vi "WPI_UtilitiesFRC LEDs.vi"(8 "error in (no error)":errorcluster, 10 "State":T1, 11 "LED Type":T2) -> (0 "error out":errorcluster, 3 "LED State":bool)   [LabVIEW 2019]
doc: "Sets the state, either on or off, of the USER1 LED or the FPGA LED on the CompactRIO device. You can define both the USER1 LED and the FPGA LED to meet the needs of your application.\n\nThis software is licensed. Open the labview\\readme\\WPI Robotics Library Open Source License.txt file for more information."
uses:
  <vilib>/Rock Robotics/SystemInterfaces/Utilities/FPGA_UtilitiesLED Source.ctl
  <vilib>/Rock Robotics/SystemInterfaces/Utilities/FPGA_UtilitiesLED State.ctl
  <vilib>/NI_Real-Time Target Support.lvlib
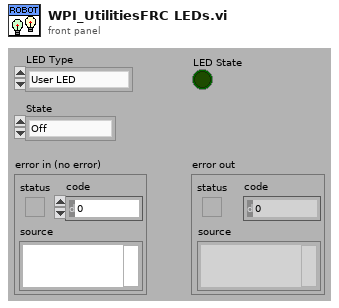
[diagram p1: front panel]
types:
  T1 = typedef "FPGA_UtilitiesLED State.ctl" = enum16{"Off", "On", "Toggle"}
  T2 = typedef "FPGA_UtilitiesLED Source.ctl" = enum16{"User LED", "FPGA LED"}
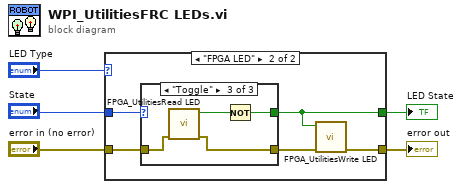
[diagram p0: block diagram]
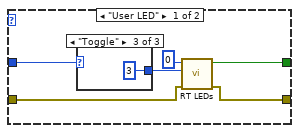
[diagram p2: hidden frame]
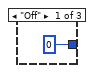
[diagram p3: hidden frame]
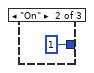
[diagram p4: hidden frame]
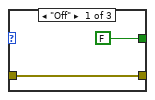
[diagram p5: hidden frame]
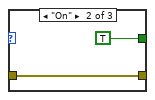
[diagram p6: hidden frame]
diagram:
  n1 = case shown="\"FPGA LED\"" "LED Type" {
    tunnel: "State" -> [w11 w19]
    tunnel: "error in (no error)" -> [w8 w16]
    tunnel: [w7 w18] -> w2
    tunnel: [w6 w17] -> w1
    frame "User LED" {
      n2 = case shown="\"Toggle\"" w11 {
        tunnel: [0 ("State") 1 ("State") 3 ("State")] -> w9
        frame "Off" {
        }
        frame "On" {
        }
        frame "Toggle" {
        }
      }
      n3 = call <vilib>:"RT LEDs.vi"("error in (no error)"=w8, "State"=w9, "LED Num"=0) -> ("error out"=w7:errorcluster, "Led State"=w6:bool)  [unwired: 3 out]
    }
    frame "FPGA LED" {
      n4 = case shown="\"Toggle\"" w19 {
        tunnel: [FALSE TRUE w27] -> w17
        tunnel: w16 -> [w20 w22 w25]
        tunnel: [w20 w22 w24] -> w15
        frame "Off" {
        }
        frame "On" {
        }
        frame "Toggle" {
          n5 = call <vilib>:"FPGA_UtilitiesRead LED.vi"("error in (no error)"=w25) -> ("error out"=w24:errorcluster, "FPGA LED"=w26:bool)  [unwired: 9 out]
          n6 = Not(x=w26) -> (.not. x?=w27:bool)
        }
      }
      n7 = call <vilib>:"FPGA_UtilitiesWrite LED.vi"("error in (no error)"=w15, "FPGA LED"=w17) -> ("error out"=w18:errorcluster)  [unwired: 9 out]
    }
  }
  "error out" <- w2
  "LED State" <- w1
